vi "SSE.vi"(7 "LabVIEW Web Service Request":refnum<class "Web Request.lvclass">=refnum, 10 "variables":string, 11 "expId":string) -> ()   [LabVIEW 2019]
uses:
  <vilib>/wsapi/Web Request.lvclass
  Configuration/Global_Configurations.vi
  <vilib>/wsapi/class/subVIs/Write Integer Session Variable.vi
panel:
  out "initTime":u32
  out "expIndex":i32
  # "Use the Web Service Request input terminal to call the VIs on the Web Services palette. Do not remove it from the connector pane unless you don't need access to the palette."
  # "Each additional control wired to the connector pane will be available as an input in the URL. To include an indicator in terminal-mode output (the default setting), it must also be wired to the connector pane."
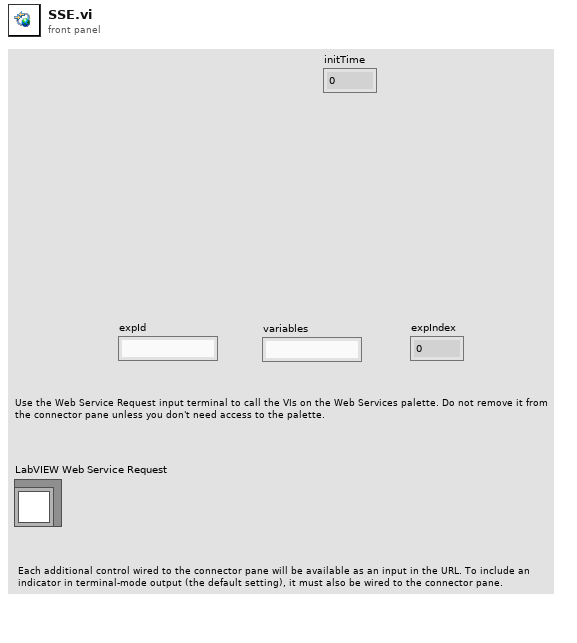
[diagram p1: front panel]
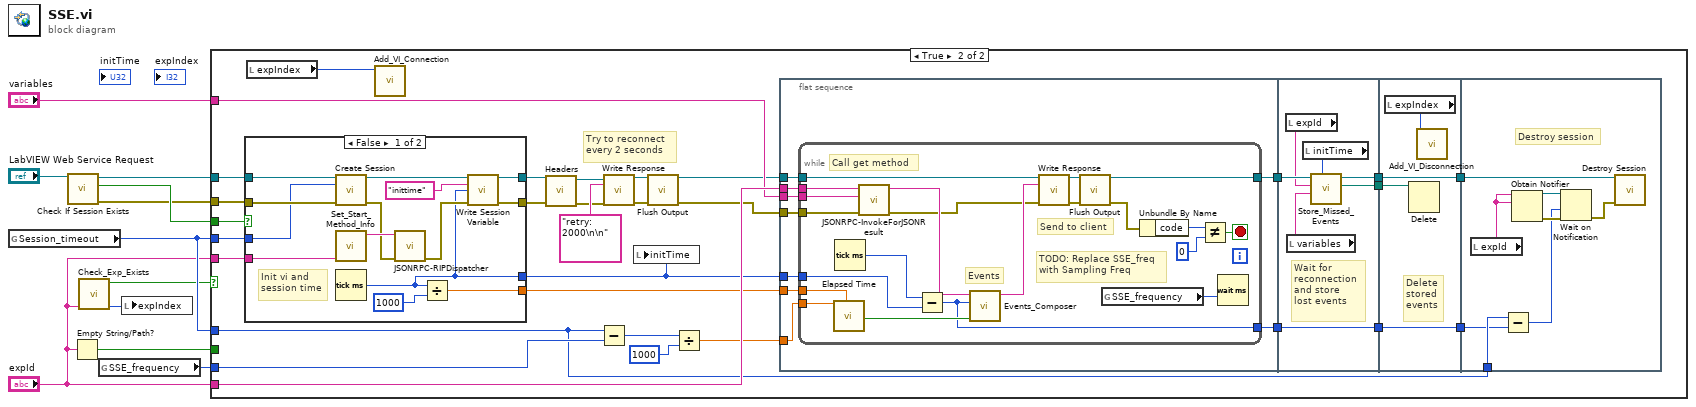
[diagram p0: block diagram]
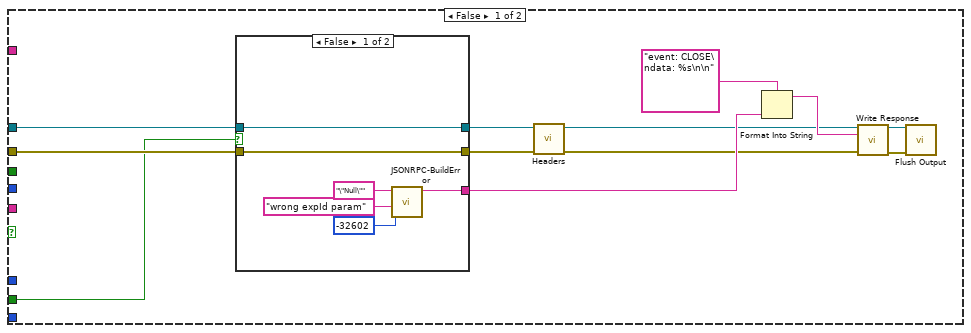
[diagram p2: hidden frame]
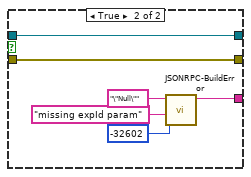
[diagram p3: hidden frame]
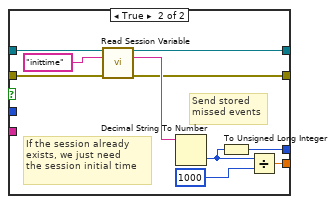
[diagram p4: hidden frame]
diagram:
  n1 = global read "Global_Configurations.vi" "Session_timeout"() -> (w9:u32)
  n2 = call <vilib>:"Check If Session Exists.vi"("LabVIEW Web Service Request"="LabVIEW Web Service Request") -> ("LabVIEW Web Service Request out"=w1:refnum<class "Web Request.lvclass">, "session exists?"=w7:bool, "error out"=w3:errorcluster)  [unwired: 12 in]
  n3 = Empty String/Path?(string/path="expId") -> (empty?=w5:bool)
  n4 = call "Check_Exp_Exists.vi"("expId"="expId") -> ("expIndex"=w2:i32, "exists"=w8:bool)  [unwired: 9 in]
  n5 = global read "Global_Configurations.vi" "SSE_frequency"() -> (w10:u32)
  n6 = local write "expIndex"(w2) -> ()
  n7 = case shown="True" w8 {
    tunnel: "expId" -> [_ w58]
    tunnel: w9 -> [_ w41]
    tunnel: w10 -> [_ w62]
    tunnel: w1 -> [w23 w60]
    tunnel: w3 -> [w22 w59]
    tunnel: "expId" -> [_ w56]
    tunnel: w7 -> [_ w38]
    tunnel: w9 -> [_ w55]
    tunnel: w5 -> [w21 _]
    tunnel: "variables" -> [_ w46]
    frame False {
      n8 = case shown="False" w21 {
        tunnel: w23 -> [w29 w31]
        tunnel: w22 -> [w28 w30]
        tunnel: [w24 w32] -> w16
        tunnel: [w29 w31] -> w15
        tunnel: [w28 w30] -> w14
        frame False {
          n9 = call "JSONRPC-BuildError.vi"("Message"="wrong expId param", "Code"=-32602, "ID"="\"Null\"") -> ("String"=w24:string)  [unwired: 8 in]
        }
        frame True {
          n10 = call "JSONRPC-BuildError.vi"("Message"="missing expId param", "Code"=-32602, "ID"="\"Null\"") -> ("String"=w32:string)  [unwired: 8 in]
        }
      }
      n11 = call "Headers.vi"("error in (no error)"=w14, "LabVIEW Web Service Request"=w15) -> ("error out"=w12:errorcluster, "LabVIEW Web Service Request out"=w13:refnum<class "Web Request.lvclass">)  [unwired: 8 in]
      n12 = Format Into String(format string="event: CLOSE\ndata: %s\n\n", w16) -> (resulting string=w20:string)  [unwired: 2 in, 1 out]
      n13 = call <vilib>:"Write Response.vi"("LabVIEW Web Service Request"=w13, "response string"=w20, "error in (no error)"=w12) -> ("LabVIEW Web Service Request out"=w18:refnum<class "Web Request.lvclass">, "error out"=w17:errorcluster)  [unwired: 11 in]
      n14 = call <vilib>:"Flush Output.vi"("LabVIEW Web Service Request"=w18, "error in (no error)"=w17) -> ()  [unwired: 12 in, 2 out]
    }
    frame True {
      # "Try to reconnect \nevery 2 seconds"
      n15 = case shown="False" w38 {
        tunnel: w60 -> [w80 w88]
        tunnel: [w68 w81] -> w53
        tunnel: w59 -> [w79 w87]
        tunnel: [w67 w86] -> w54
        tunnel: w55 -> [w78 _]
        tunnel: w56 -> [w77 _]
        tunnel: [w69 w84] -> w57
        tunnel: [w70 w83] -> w39
        frame False {
          # "Init vi and \nsession time"
          n16 = call <vilib>:"Create Session.vi"("LabVIEW Web Service Request"=w80, "timeout (60000 msec)"=w78, "error in (no error)"=w79) -> ("LabVIEW Web Service Request out"=w73:refnum<class "Web Request.lvclass">, "error out"=w75:errorcluster)  [unwired: 10 in, 1 out]
          n17 = call "Set_Start_Method_Info.vi"("expId"=w77) -> ("String"=w76:string)  [unwired: 10 in]
          n18 = Tick Count (ms)() -> (millisecond timer value=w70:u32)
          n19 = call "JSONRPC-RIPDispatcher.vi"("error in"=w75, "input string"=w76) -> ("error out"=w72:errorcluster)  [unwired: 8 in, 1 out]
          n20 = Divide(x=w70, y=u32 1000) -> (x/y=w69:dbl)
          n21 = call-poly <vilib>:"Write Session Variable.vi"("LabVIEW Web Service Request"=w73, "key"="inittime", "value"=w70, "error in (no error)"=w72) -> ("LabVIEW Web Service Request out"=w68:refnum<class "Web Request.lvclass">, "error out"=w67:errorcluster)  [unwired: 8 in, 2 out]
        }
        frame True {
          # "Send stored \nmissed events"
          # "If the session already exists, we just need \nthe session initial time"
          n22 = call <vilib>:"Read Session Variable.vi"("LabVIEW Web Service Request"=w88, "key"="inittime", "error in (no error)"=w87) -> ("LabVIEW Web Service Request out"=w81:refnum<class "Web Request.lvclass">, "value"=w90:string, "error out"=w86:errorcluster)  [unwired: 10 in]
          n23 = Decimal String To Number(string=w90) -> (number=w82:i32)  [unwired: 2 in, 1 out]
          n24 = To Unsigned Long Integer(number=w82) -> (unsigned 32bit integer=w83:u32)
          n25 = Divide(x=w82, y=u32 1000) -> (x/y=w84:dbl)
        }
      }
      n26 = local read "expIndex"() -> (w50:i32)
      n27 = call "Add_VI_Connection.vi"("expIndex"=w50) -> ()  [unwired: 11 in]
      n28 = call "Headers.vi"("error in (no error)"=w54, "LabVIEW Web Service Request"=w53) -> ("error out"=w51:errorcluster, "LabVIEW Web Service Request out"=w52:refnum<class "Web Request.lvclass">)  [unwired: 8 in]
      n29 = Subtract(x=w41, y=w62) -> (x-y=w61:u32)
      n30 = call <vilib>:"Write Response.vi"("LabVIEW Web Service Request"=w52, "response string"="retry: 2000\n\n", "error in (no error)"=w51) -> ("LabVIEW Web Service Request out"=w66:refnum<class "Web Request.lvclass">, "error out"=w65:errorcluster)  [unwired: 11 in]
      n31 = local write "initTime"(w39) -> ()
      n32 = call <vilib>:"Flush Output.vi"("LabVIEW Web Service Request"=w66, "error in (no error)"=w65) -> ("LabVIEW Web Service Request out"=w37:refnum<class "Web Request.lvclass">, "error out"=w36:errorcluster)  [unwired: 12 in]
      n33 = Divide(x=w61, y=u32 1000) -> (x/y=w47:dbl)
      n34 = flat-sequence {
        tunnel: w37 -> [w99]
        tunnel: w36 -> [w98]
        tunnel: w58 -> [w97]
        tunnel: w57 -> [w96]
        tunnel: w47 -> [w95]
        tunnel: w39 -> [w94]
        tunnel: [w93] -> w49
        tunnel: w46 -> [w92]
        tunnel: [w91] -> w44
        tunnel: [w125] -> w48
        tunnel: w49 -> [w126]
        tunnel: [w127] -> w45
        tunnel: w44 -> [w127]
        tunnel: [w122] -> w40
        tunnel: w48 -> [w131]
        tunnel: [w131] -> w43
        tunnel: [w129] -> w42
        tunnel: w45 -> [w129]
        tunnel: w40 -> [w128]
        tunnel: w43 -> [w136]
        tunnel: w42 -> [w133]
        tunnel: w41 -> [w134]
        frame #0 {
          n35 = while {
            tunnel: w99 -> [w109]
            tunnel: w98 -> [w114]
            tunnel: w97 -> [w115]
            tunnel: w96 -> [w106]
            tunnel: w95 -> [w108]
            tunnel: w94 -> [w104]
            tunnel: [w103] -> w93
            tunnel: w92 -> [w101]
            tunnel: [w100] -> w91
            stop <- w116 stop-if-true
            # "TODO: Replace SSE_freq\nwith Sampling Freq"
            # "Send to client"
            # "Events"
            # "Call get method"
            n36 = call "Elapsed Time"("Time Target (s)"=w108, "Set Start Time (s)"=w106) -> ("Time has Elapsed"=w107:bool)  [unwired: 10 in, 7 out]
            n37 = Tick Count (ms)() -> (millisecond timer value=w105:u32)
            n38 = call "JSONRPC-InvokeForJSONResult.vi"("error in"=w114, "variables"=w101, "expid"=w115) -> ("error out"=w110:errorcluster, "response"=w112:string)  [unwired: 7 in]
            n39 = Subtract(x=w105, y=w104) -> (x-y=w100:u32)
            n40 = call "Events_Composer.vi"("hearbeat"=w107, "time"=w100, "responsein"=w112) -> ("responseout"=w113:string)  [unwired: 8 in]
            n41 = call <vilib>:"Write Response.vi"("LabVIEW Web Service Request"=w109, "response string"=w113, "error in (no error)"=w110) -> ("LabVIEW Web Service Request out"=w119:refnum<class "Web Request.lvclass">, "error out"=w120:errorcluster)  [unwired: 11 in]
            n42 = call <vilib>:"Flush Output.vi"("LabVIEW Web Service Request"=w119, "error in (no error)"=w120) -> ("LabVIEW Web Service Request out"=w103:refnum<class "Web Request.lvclass">, "error out"=w102:errorcluster)  [unwired: 12 in]
            n43 = global read "Global_Configurations.vi" "SSE_frequency"() -> (w111:u32)
            n44 = Unbundle By Name(w102) -> ("code"=w118:i32)
            n45 = Not Equal?(x=w118, y=0) -> (x != y?=w116:bool)
            n46 = Wait (ms)(milliseconds to wait=w111) -> ()  [unwired: 1 out]
          }
        }
        frame #1 {
          # "Wait for\nreconnection\nand store\nlost events"
          n47 = local read "expId"() -> (w124:string)
          n48 = local read "variables"() -> (w123:string)
          n49 = local read "initTime"() -> (w121:u32)
          n50 = call "Store_Missed_Events.vi"("initTime"=w121, "variables"=w123, "expId"=w124, "LabVIEW Web Service Request"=w126) -> ("path"=w122:path, "LabVIEW Web Service Request out"=w125:refnum<class "Web Request.lvclass">)  [unwired: 6 in]
        }
        frame #2 {
          # "Delete \nstored \nevents"
          n51 = local read "expIndex"() -> (w130:i32)
          n52 = Delete(path (use dialog)=w128) -> ()  [unwired: 4 in, 3 out]
          n53 = call "Add_VI_Disconnection.vi"("expIndex"=w130) -> ()  [unwired: 11 in]
        }
        frame #3 {
          # "Destroy session"
          n54 = local read "expId"() -> (w135:string)
          n55 = Subtract(x=w134, y=w133) -> (x-y=w132:u32)
          n56 = Obtain Notifier(name (unnamed)=w135, notification data type=w135) -> (notifier out=w139:refnum<notifier>, error out=w138:errorcluster)  [unwired: 2 in, 1 out]
          n57 = Wait on Notification(notifier=w139, timeout in ms (-1)=w132, error in (no error)=w138) -> (error out=w137:errorcluster)  [unwired: 1 in, 3 out]
          n58 = call <vilib>:"Destroy Session.vi"("LabVIEW Web Service Request"=w136, "error in (no error)"=w137) -> ()  [unwired: 12 in, 2 out]
        }
      }
    }
  }
